vi "read inputs.vi"(8 "error in":errorcluster, 10 "Timeout (ms)":i32=-1, 11 "profibus reference":T2) -> (0 "error out":errorcluster, 1 "diagnostics":T1[](array[typedef]), 2 "inputs":T1[](array[typedef]), 3 "profibus reference out":T2)   [LabVIEW 2013, in "dynamic profibus.lvlib"]
uses:
  dynamic profibus.lvlib
  fpga reference.ctl
  input data.ctl
  read input state machine.ctl
  profibus master transmit header.ctl
  <vilib>/rvi/interface/common/niFpgaWaitOnOcc.vi
  <vilib>/Utility/error.llb/Error Cluster From Error Code.vi
  <vilib>/rvi/errors/niLvFpgaAdjustHostInterfaceError.vi
  <vilib>/rvi/interface/nirviMethod/nirviMethod.xnode
  <vilib>/FPGAPlugInAG/Dynamic/niLvFpga_ReadFifo_Dynamic.vi
  <vilib>/rvi/errors/niLvFpgaMergeErrorWithErrorCode.vi
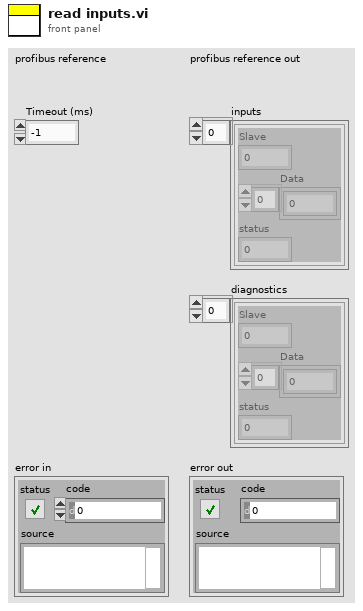
[diagram p1: front panel]
types:
  T1 = typedef "dynamic profibus.lvlib/input data.ctl" = cluster{"Slave":u8, "Data":u8[], "status":u8}
  T2 = typedef "dynamic profibus.lvlib/fpga reference.ctl" = refnum<k20>
  T3 = typedef "dynamic profibus.lvlib/read input state machine.ctl" = enum16{"Wait for first data", "Check timeout", "Read Length"}
  T4 = typedef "profibus master transmit header.ctl" = enum8{"Input", "Diagnostic"}
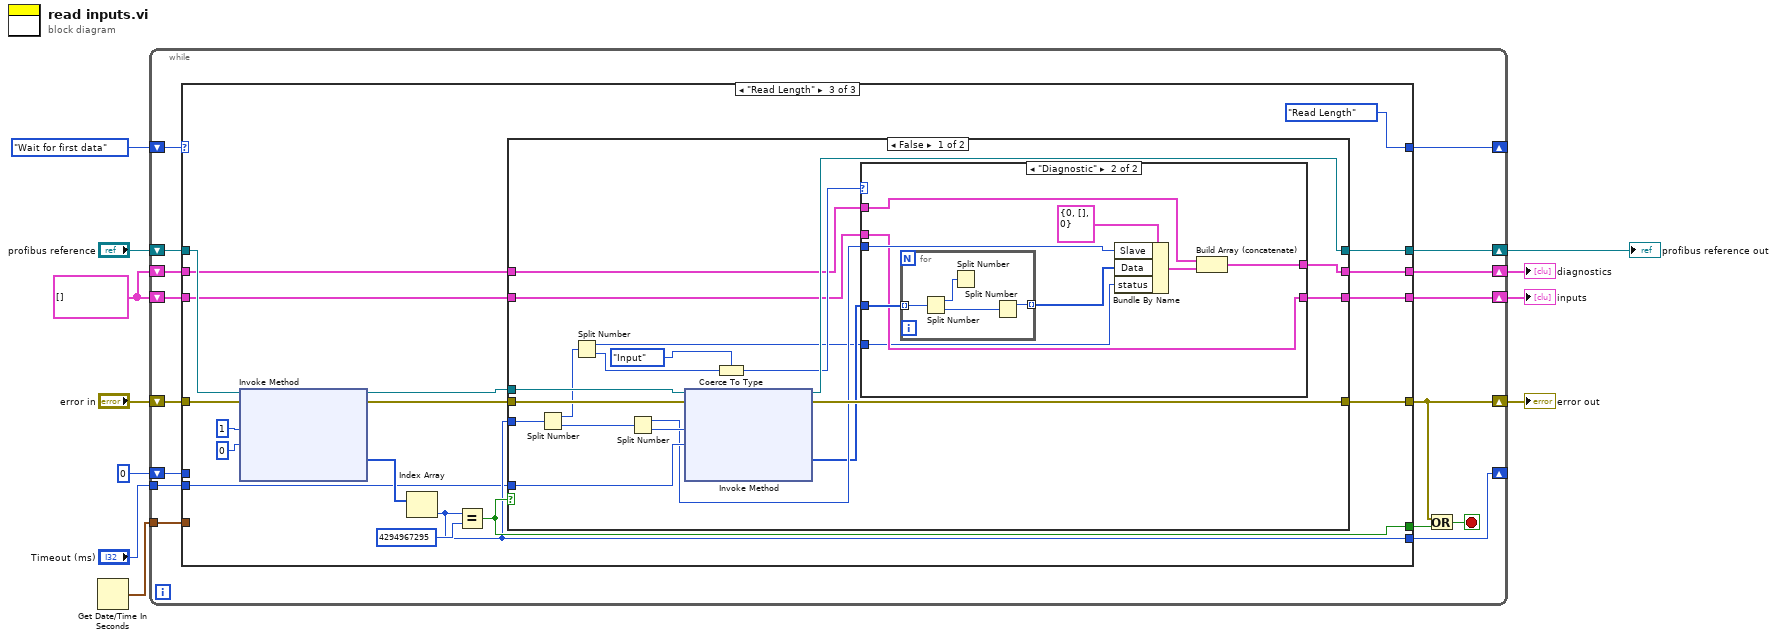
[diagram p0: block diagram]
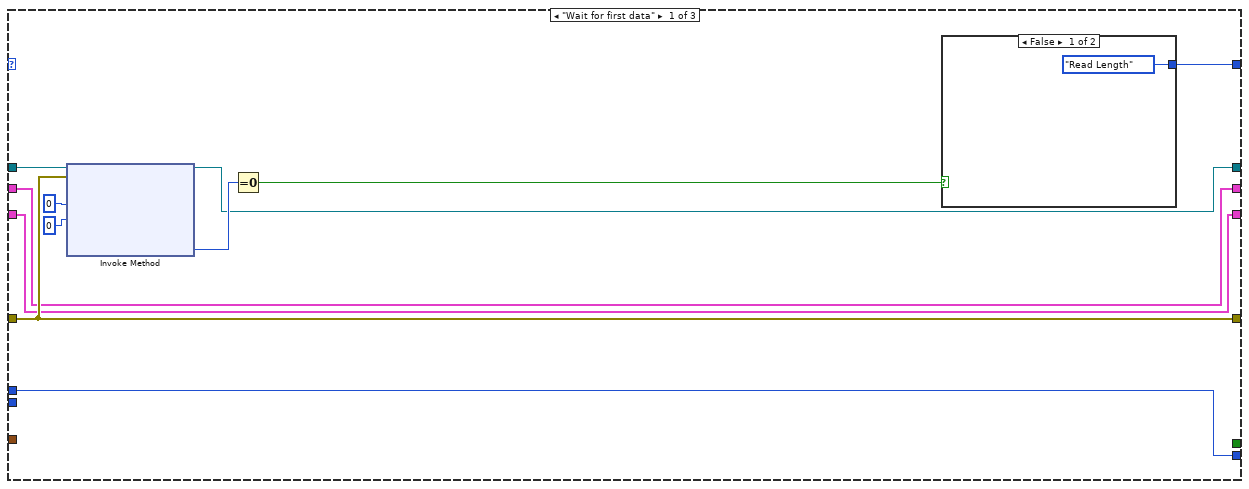
[diagram p2: hidden frame]
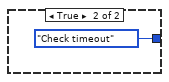
[diagram p3: hidden frame]
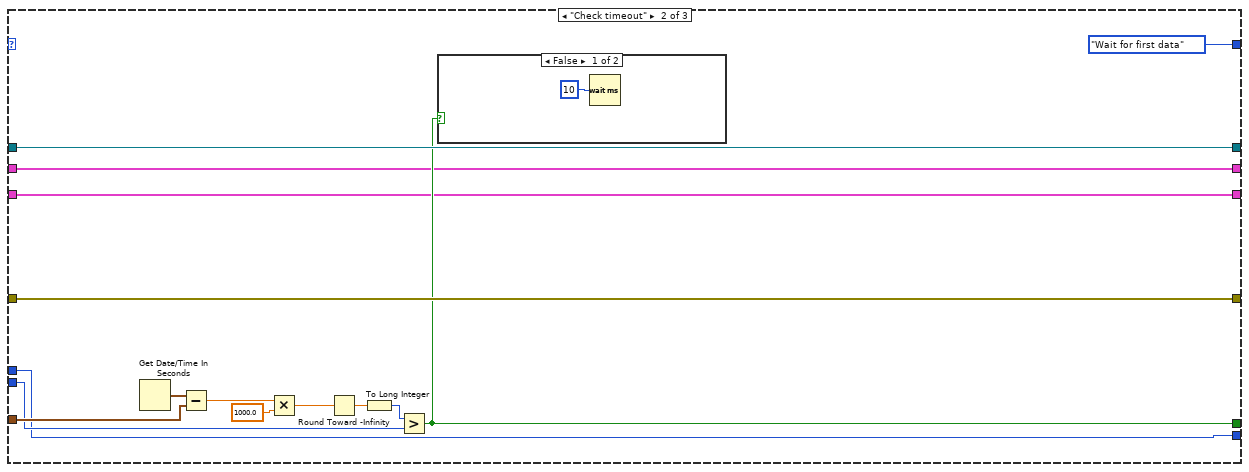
[diagram p4: hidden frame]
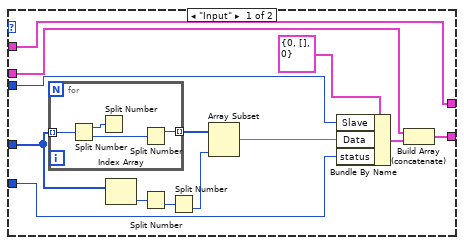
[diagram p6: hidden frame]
diagram:
  w3 = T1[] []
  n1 = Get Date/Time In Seconds() -> (seconds since 1Jan1904=w6:timestamp)
  n2 = while {
    shift-right: [w24] -> _
    shift-left: read_input_state_machine."Wait for first data" -> [w27]
    shift-right: [w23] -> w8
    shift-left: "profibus reference" -> [w25]
    shift-right: [w21] -> w7
    shift-left: "error in" -> [w26]
    tunnel: w6 -> [w20]
    tunnel: "Timeout (ms)" -> [w19]
    shift-right: [w17] -> _
    shift-left: u32 0 ("Number of Elements") -> [w16]
    shift-right: [w15] -> w2
    shift-left: w3 -> [w14]
    shift-right: [w12] -> w1
    shift-left: w3 -> [w13]
    stop <- w22 stop-if-true
    n3 = case shown="\"Read Length\"" w27 {
      tunnel: w26 -> [w31 w54 w73]
      tunnel: w25 -> [w36 w55 w74]
      tunnel: [w33 read_input_state_machine."Wait for first data" read_input_state_machine."Read Length"] -> w24
      tunnel: [w32 w55 w64] -> w23
      tunnel: [w31 w54 w66] -> w21
      tunnel: w20 -> [_ w51 _]
      tunnel: w19 -> [_ w45 w61]
      tunnel: [_ w44 w63] -> w18
      tunnel: [w30 w43 w62] -> w17
      tunnel: w16 -> [w30 w43 _]
      tunnel: [w29 w42 w60] -> w15
      tunnel: w14 -> [w29 w42 w59]
      tunnel: w13 -> [w28 w41 w58]
      tunnel: [w28 w41 w57] -> w12
      frame "Wait for first data" {
        n4 = xnode "Invoke Method"("FPGA VI Reference In"=w36, "error in"=w31, "Number of Elements"=u32 0, "Timeout (ms)"=0) -> ("FPGA VI Reference Out"=w32:T2, "Elements Remaining"=w35:u32)  [unwired: 2 out]
        n5 = Equal To 0?(x=w35) -> (x = 0?=w34:bool)
        n6 = case shown="False" w34 {
          tunnel: [read_input_state_machine."Read Length" read_input_state_machine."Check timeout"] -> w33
          frame False {
          }
          frame True {
          }
        }
      }
      frame "Check timeout" {
        n7 = Get Date/Time In Seconds() -> (seconds since 1Jan1904=w52:timestamp)
        n8 = Subtract(x=w52, y=w51) -> (x-y=w50:dbl)
        n9 = Multiply(x=w50, y=1000.0) -> (x*y=w48:dbl)
        n10 = Round Toward -Infinity(1:w48) -> (0:w47:dbl)
        n11 = To Long Integer(number=w47) -> (32bit integer=w46:i32)
        n12 = Greater?(x=w46, y=w45) -> (0:w44:bool)
        n13 = case shown="False" w44 {
          frame False {
            n14 = Wait (ms)(milliseconds to wait=u32 10) -> ()  [unwired: 1 out]
          }
          frame True {
          }
        }
      }
      frame "Read Length" {
        n15 = xnode "Invoke Method"("FPGA VI Reference In"=w74, "error in"=w73, "Number of Elements"=u32 1, "Timeout (ms)"=0) -> ("FPGA VI Reference Out"=w65:T2, "error out"=w70:errorcluster, "Data"=w69:u32[])  [unwired: 1 out]
        n16 = Index Array(array=w69) -> (element=w62:u32)  [unwired: 1 in]
        n17 = Equal?(x=w62, y=u32 4294967295 ("Element")) -> (x = y?=w63:bool)
        n18 = case shown="False" w63 {
          tunnel: w70 -> [w93 w126]
          tunnel: [w92 w126] -> w66
          tunnel: w65 -> [w91 w127]
          tunnel: [w90 w127] -> w64
          tunnel: w62 -> [w87 _]
          tunnel: w61 -> [w86 _]
          tunnel: [w79 w124] -> w60
          tunnel: w59 -> [w78 w124]
          tunnel: w58 -> [w77 w125]
          tunnel: [w76 w125] -> w57
          frame False {
            n19 = Split Number(x=w87) -> (hi(x)=w88:u16, lo(x)=w89:u16)
            n20 = Split Number(x=w88) -> (hi(x)=w75:u8, lo(x)=w81:u8)
            n21 = Split Number(x=w89) -> (hi(x)=w84:u8, lo(x)=w85:u8)
            n22 = xnode "Invoke Method"("FPGA VI Reference In"=w91, "error in"=w93, "Number of Elements"=w85, "Timeout (ms)"=w86) -> ("FPGA VI Reference Out"=w90:T2, "error out"=w92:errorcluster, "Data"=w80:u32[])  [unwired: 1 out]
            n23 = Coerce To Type(0:w81, 1:profibus_master_transmit_header."Input") -> (2:w82:T4)
            n24 = case shown="\"Diagnostic\"" w82 {
              tunnel: w84 -> [w104 w117]
              tunnel: w80 -> [w99 w119]
              tunnel: [w101 w115] -> w79
              tunnel: w78 -> [w103 w115]
              tunnel: w77 -> [w102 w114]
              tunnel: [w102 w113] -> w76
              tunnel: w75 -> [w94 w111]
              frame "Input" {
                n25 = for {
                  tunnel: w99 -> [w110] mode=indexing
                  tunnel: [w107] -> w105 mode=indexing
                  n26 = Split Number(x=w110) -> (hi(x)=w109:u16, lo(x)=w108:u16)
                  n27 = Split Number(x=w109) -> ()  [unwired: 2 out]
                  n28 = Split Number(x=w108) -> (hi(x)=w107:u8)  [unwired: 1 out]
                }
                n29 = Index Array(array=w99) -> (element=w97:u32)  [unwired: 1 in]
                n30 = Split Number(x=w97) -> (lo(x)=w98:u16)  [unwired: 1 out]
                n31 = Split Number(x=w98) -> (lo(x)=w95:u8)  [unwired: 1 out]
                n32 = Array Subset(array=w105, length=w95) -> (w96:u8[])  [unwired: 1 in]
                n33 = Bundle By Name(cluster=T1 {"Slave"=0, "Data"=[], "status"=0} ("Output Data"), "Slave"=w104, "Data"=w96, "status"=w94) -> (w100:T1)
                n34 = Build Array (concatenate)(w103, w100) -> (w101:T1[])
              }
              frame "Diagnostic" {
                n35 = for {
                  tunnel: w119 -> [w123] mode=indexing
                  tunnel: [w120] -> w118 mode=indexing
                  n36 = Split Number(x=w123) -> (hi(x)=w122:u16, lo(x)=w121:u16)
                  n37 = Split Number(x=w122) -> ()  [unwired: 2 out]
                  n38 = Split Number(x=w121) -> (hi(x)=w120:u8)  [unwired: 1 out]
                }
                n39 = Bundle By Name(cluster=T1 {"Slave"=0, "Data"=[], "status"=0} ("Output Data"), "Slave"=w117, "Data"=w118, "status"=w111) -> (w116:T1)
                n40 = Build Array (concatenate)(w114, w116) -> (w113:T1[])
              }
            }
          }
          frame True {
          }
        }
      }
    }
    n41 = Or(x=w21, y=w18) -> (x .or. y?=w22:bool)
  }
  "error out" <- w7
  "profibus reference out" <- w8
  "inputs" <- w2
  "diagnostics" <- w1
